vi "CreateUINetworkStreamReader.vi"(8 "ErrorIn":errorcluster, 10 "ReaderName":string="Win/Data", 11 "IPAddress":string) -> (0 "ErrorOut":errorcluster, 3 "reader endpoint":refnum<k21>)   [LabVIEW 2018]
uses:
  Controls/Enums/StreamReceiveStates.ctl
  Controls/Clusts/StreamReceiveClust.ctl
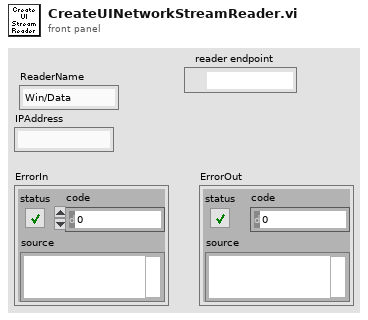
[diagram p1: front panel]
types:
  T1 = typedef "StreamReceiveStates.ctl" = enum16{"Rcv:Init", "Rcv:Read", "Rcv:Log", "Rcv:FromMast", "Rcv:FromSlav"}
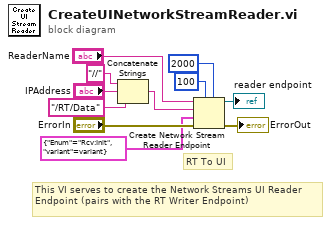
[diagram p0: block diagram]
diagram:
  # "This VI serves to create the Network Streams UI Reader Endpoint (pairs with the RT Writer Endpoint)"
  # "RT To UI"
  n1 = Concatenate Strings("//" ("string"), "IPAddress", "/RT/Data" ("Name")) -> (w6:string)
  n2 = Create Network Stream Reader Endpoint(5:2000 ("writer buffer size"), 7:100 ("writer buffer size"), 8:"ErrorIn", 9:cluster{"Enum":T1, "variant":variant} {"Enum"=enum."Rcv:Init", "variant"=variant}, 10:w6, 11:"ReaderName") -> (0:→"ErrorOut":errorcluster, 3:→"reader endpoint":refnum<k21>)  [unwired: 1 in]
